vi "v0 Elevador con maquina de casos.vi"() -> ()   [LabVIEW 2018]
panel:
  out "Piso actual":i32
  in  "stop":bool
  out "Down":bool
  out "Up":bool
  in  "P3_A":bool
  in  "P2_A":bool
  in  "P1_A":bool
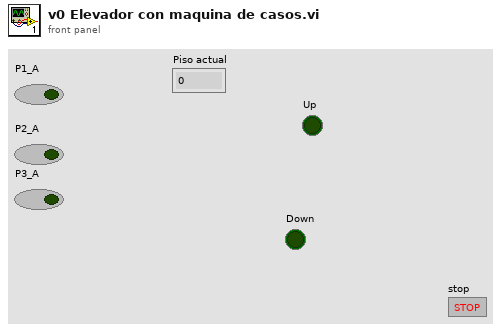
[diagram p1: front panel]
types:
  T1 = enum16{"E1", "E2", "E3", "E4", "E5", "E6", "E7", "E8", "E9", "E10", ""}
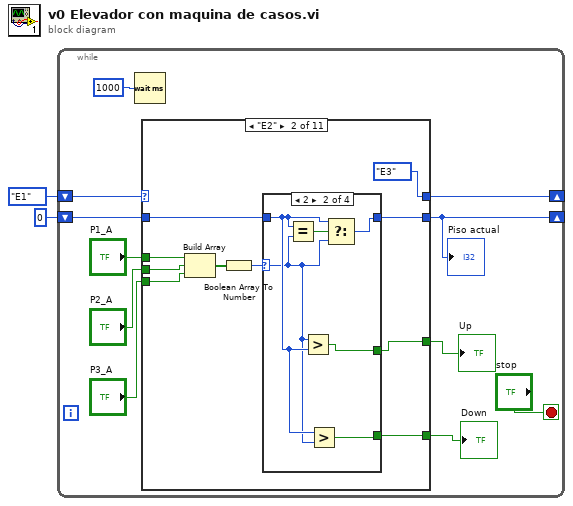
[diagram p0: block diagram]
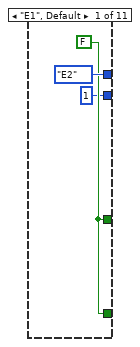
[diagram p2: hidden frame]
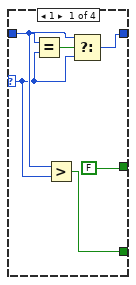
[diagram p3: hidden frame]
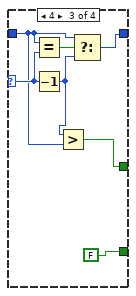
[diagram p4: hidden frame]
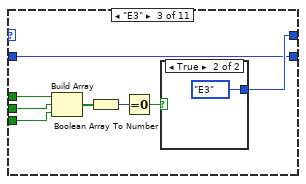
[diagram p6: hidden frame]
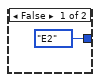
[diagram p7: hidden frame]
diagram:
  n1 = while {
    shift-right: [w10] -> _
    shift-left: T1."E1" ("Enum") -> [w13]
    shift-right: [w3] -> _
    shift-left: 0 -> [w4]
    stop <- "stop" stop-if-true
    n2 = Wait (ms)(milliseconds to wait=u32 1000) -> ()  [unwired: 1 out]
    n3 = case shown="\"E2\"" w13 {
      tunnel: [T1."E2" ("Enum 2") T1."E3" ("Enum 2") w48 _ _ _ _ _ _ _ _] -> w10
      tunnel: "P1_A" -> [_ w25 w54 _ _ _ _ _ _ _ _]
      tunnel: "P2_A" -> [_ w24 w53 _ _ _ _ _ _ _ _]
      tunnel: "P3_A" -> [_ w23 w52 _ _ _ _ _ _ _ _]
      tunnel: [w15 w18 _ _ _ _ _ _ _ _ _] -> w6
      tunnel: [w15 w17 _ _ _ _ _ _ _ _ _] -> w5
      tunnel: w4 -> [_ w19 w47 _ _ _ _ _ _ _ _]
      tunnel: [1 w20 w47 _ _ _ _ _ _ _ _] -> w3
      frame "E1", Default {
        w15 = FALSE
      }
      frame "E2" {
        n4 = Build Array(w25, w24, w23) -> (w22:bool[])
        n5 = Boolean Array To Number(Boolean array=w22) -> (number=w21:u32)
        n6 = case shown="2" w21 {
          selector: w21 -> [w28 w34 w42 _]
          tunnel: [w31 w37 w44 w46] -> w20
          tunnel: w19 -> [w29 w35 w41 w46]
          tunnel: [FALSE w36 w40 _] -> w18
          tunnel: [w27 w33 FALSE _] -> w17
          frame 1 {
            n7 = Equal?(x=w29, y=w28) -> (x = y?=w32:bool)
            n8 = Greater?(x=w29, y=w28) -> (0:w27:bool)
            n9 = Select(t=w29, s=w32, f=w28) -> (s? t:f=w31:u32)
          }
          frame 2 {
            n10 = Equal?(x=w35, y=w34) -> (x = y?=w38:bool)
            n11 = Greater?(x=w34, y=w35) -> (0:w36:bool)
            n12 = Greater?(x=w35, y=w34) -> (0:w33:bool)
            n13 = Select(t=w35, s=w38, f=w34) -> (s? t:f=w37:u32)
          }
          frame 4 {
            n14 = Equal?(x=w41, y=w42) -> (x = y?=w45:bool)
            n15 = Decrement(x=w42) -> (x-1=w39:u32)
            n16 = Greater?(x=w39, y=w41) -> (0:w40:bool)
            n17 = Select(t=w41, s=w45, f=w39) -> (s? t:f=w44:u32)
          }
          frame 0, Default {
          }
        }
      }
      frame "E3" {
        n18 = Build Array(w54, w53, w52) -> (w51:bool[])
        n19 = Boolean Array To Number(Boolean array=w51) -> (number=w50:u32)
        n20 = Equal To 0?(x=w50) -> (x = 0?=w49:bool)
        n21 = case shown="True" w49 {
          tunnel: [T1."E2" ("Enum 2") T1."E3" ("Enum 2")] -> w48
          frame False {
          }
          frame True {
          }
        }
      }
      frame "E4" {
      }
      frame "E5" {
      }
      frame "E6" {
      }
      frame "E7" {
      }
      frame "E8" {
      }
      frame "E9" {
      }
      frame "E10" {
      }
      frame "" {
      }
    }
    "Up" <- w6
    "Down" <- w5
    "Piso actual" <- w3
  }
